vi "Read Attributes.vi"(11 "Return Microgrid State Msg":refnum<class "Return Microgrid State Msg.lvclass">) -> (2 "Payload":cluster{"Microgrid State":T1})   [LabVIEW 2018, in "EMS Core.lvlib" / "Return Microgrid State Msg.lvclass"]
uses:
  Return Microgrid State Msg.lvclass
  EMS/Controls/Microgrid State.ctl
  Return Microgrid State Msg.lvclass/Return Microgrid State Msg.ctl
  EMS/EMS.lvclass
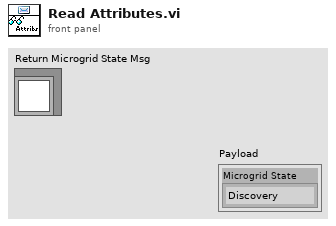
[diagram p1: front panel]
types:
  T1 = typedef "EMS Core.lvlib/EMS.lvclass/Microgrid State.ctl" = enum16{"Discovery", "Commissioning", "Activation", "Blackstart", "OnGrid", "OffGrid", "Island", "Resynchronization", "Manual", "Shutdown", "Stop"}
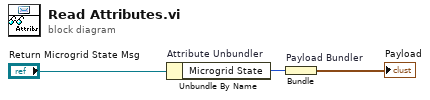
[diagram p0: block diagram]
diagram:
  n1 = Unbundle By Name "Attribute Unbundler"("Return Microgrid State Msg") -> ("Microgrid State"=w1:T1)
  n2 = Bundle "Payload Bundler"("Microgrid State"=w1) -> (→"Payload":cluster{"Microgrid State":T1})  [unwired: 1 in]
